vi "myRIO_BRig_RT_dataLC_init_details.vi"() -> (1 "output_dataSize":i32=30, 2 "output_dataName":string="dataExp")   [LabVIEW 2014]
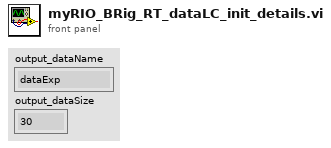
[diagram p1: front panel]
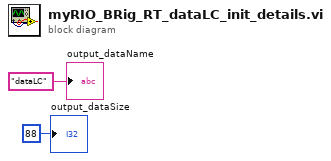
[diagram p0: block diagram]
diagram:
  "output_dataName" <- "dataLC"
  "output_dataSize" <- 88
